vi "Bytes To GBs.vi"(10 "Bytes":i64) -> (2 "GB":dbl)   [LabVIEW 2024]
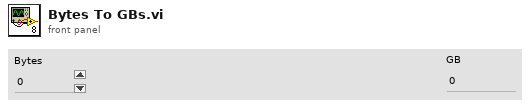
[diagram p1: front panel]
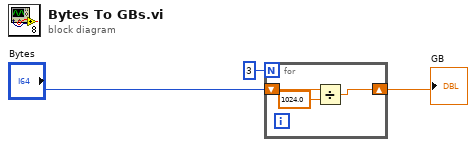
[diagram p0: block diagram]
diagram:
  n1 = for {
    N: 3 -> [_]
    shift-right: [w5] -> w1
    shift-left: "Bytes" -> [w6]
    n2 = Divide(x=w6, y=1024.0) -> (x/y=w5:dbl)
  }
  "GB" <- w1
